vi "Query Instrument Model If Exists.vi"(6 "Regular Expression":string="^\\s*(Agilent|Keysight)\\s+Technologies\\s*\\,", 7 "Models Array":string[](array[string])=["E4404A", "E4446A"], 8 "error in (no error)":errorcluster, 11 "VISA resource name":refnum<visa-resource-name>) -> (0 "Error Out":errorcluster, 2 "ID Match":bool, 4 "*IDN? Response":string)   [LabVIEW 2015]
doc: "VI will return an error condition in Error cluster if instrument model is not found."
uses:
  <vilib>/regexp/Match Regular Expression.xnode
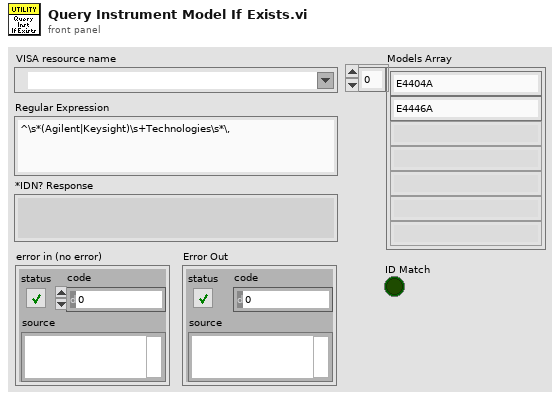
[diagram p1: front panel]
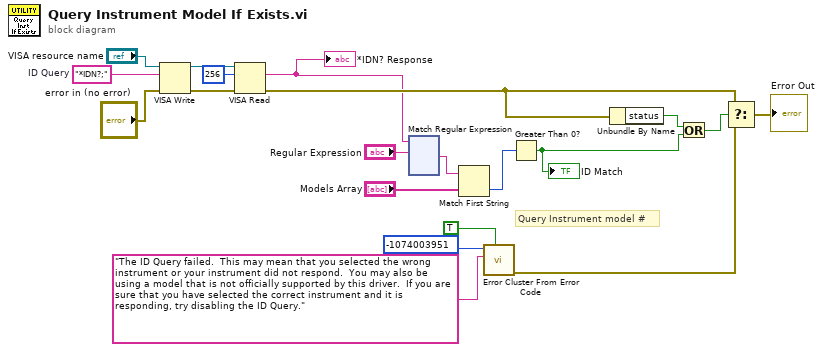
[diagram p0: block diagram]
diagram:
  w17 = "*IDN?;"  # ID Query
  # "Query Instrument model #"
  n1 = VISA Write(VISA resource name="VISA resource name", write buffer=w17, error in (no error)="error in (no error)") -> (VISA resource name out=w20:refnum<visa-resource-name>, error out=w19:errorcluster)  [unwired: 1 out]
  n2 = VISA Read(VISA resource name=w20, byte count=u32 256, error in (no error)=w19) -> (read buffer=w6:string, error out=w12:errorcluster)  [unwired: 2 out]
  "*IDN? Response" <- w6
  n3 = xnode "Match Regular Expression"("input string"=w6, "regular expression"="Regular Expression") -> ("after match"=w5:string)  [unwired: 4 in, 4 out]
  n4 = Match First String(2:"Models Array", 3:w5) -> (0:w7:i32)  [unwired: 1 out]
  n5 = call <vilib>:"Error Cluster From Error Code.vi"("show call chain? (False)"=TRUE, "error message (\"\")"="The ID Query failed.  This may mean that you selected the wrong instrument or your instrument did not respond.  You may also be using a model that is not officially supported by this driver.  If you are sure that you have selected the correct instrument and it is responding, try disabling the ID Query." ("Source (VI Name)"), "error code (0)"=-1074003951 ("Code")) -> ("error out"=w16:errorcluster)  [unwired: 1 in, 5 out]
  n6 = Greater Than 0?(x=w7) -> (x > 0?=w10:bool)
  "ID Match" <- w10
  n7 = Unbundle By Name(w12) -> ("status"=w11:bool)
  n8 = Or(x=w11, y=w10) -> (x .or. y?=w9:bool)
  n9 = Select(t=w12, s=w9, f=w16) -> (s? t:f=→"Error Out":errorcluster)
